vi "Calculate Ext Parameters.vi"(8 "error in":errorcluster, 11 "CRDS in":refnum<class "CRDS.lvclass">) -> (0 "error out":errorcluster, 2 "CRDS Data out":refnum<class "CRDS Data.lvclass">, 3 "CRDS out":refnum<class "CRDS.lvclass">)   [LabVIEW 2011, in "CRDS.lvclass"]
uses:
  CRDS.lvclass
  Data Class/Main Class/CRDS Data.lvclass
  Data Class/Cell Class/CRDS Cell Data.lvclass
  Cell Class/CRDS Cell.lvclass
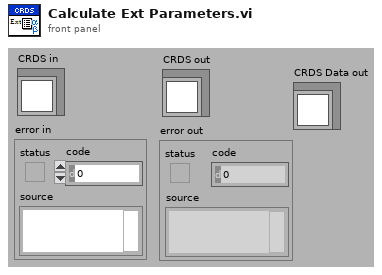
[diagram p1: front panel]
types:
  T1 = typedef "chDescr.ctl" = enum16{"Ref", "Dry", "60%", "90%"}
  T2 = typedef "las_lambda.ctl" = enum16{"Red", "Blue", "Green"}
  T3 = typedef "Get Tau Method.ctl" = enum8{"DFT-1", "DFT-5", "LRS"}
  T4 = cluster{"CalType":T3, "errorCalOn":bool, "lambda":sgl, "optTimeConst":sgl}
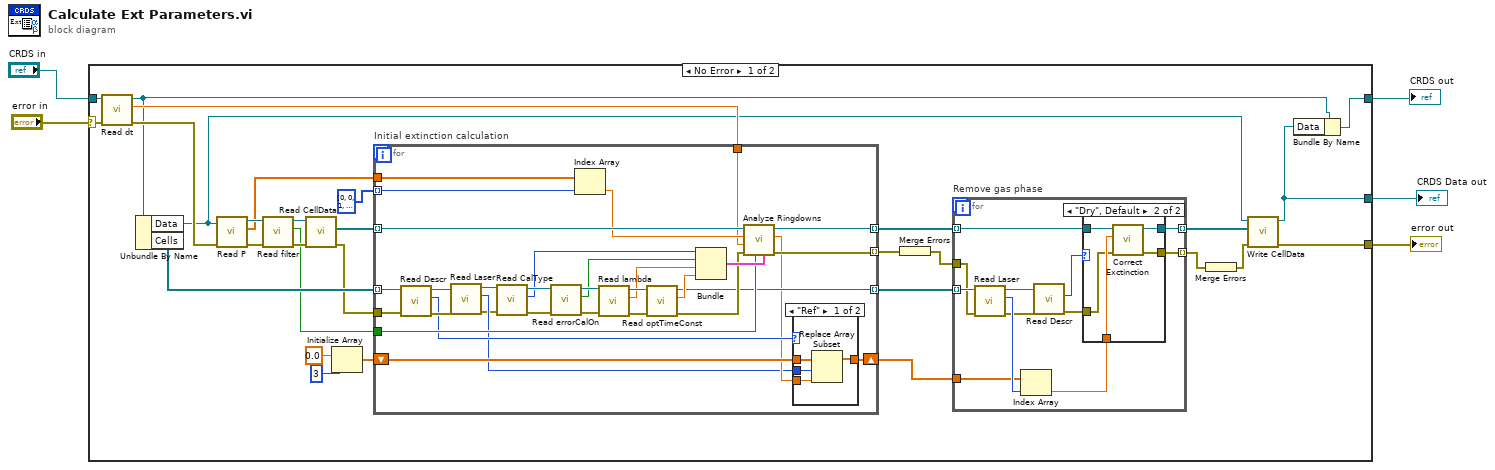
[diagram p0: block diagram]
diagram:
  n1 = case shown="No Error" "error in" {
    selector: "error in" -> [w23 w93]
    tunnel: [w10 w93] -> w4
    tunnel: [w8 w92] -> w2
    tunnel: "CRDS in" -> [w25 w92]
    tunnel: [w6 _] -> w1
    frame No Error {
      n2 = call "Read dt.vi"("error in (no error)"=w23, "CRDS in"=w25) -> ("error out"=w22:errorcluster, "dt"=w24:sgl, "CRDS out"=w9:refnum<class "CRDS.lvclass">)  [unwired: 7 in]
      n3 = Unbundle By Name(w9) -> ("Data"=w7:refnum<class "CRDS Data.lvclass">, "Cells"=w34:refnum<class "CRDS Cell.lvclass">[])
      n4 = call "Read P.vi"("error in (no error)"=w22, "CRDS Data in"=w7) -> ("error out"=w29:errorcluster, "P"=w26:sgl[], "CRDS Data out"=w28:refnum<class "CRDS Data.lvclass">)  [unwired: 7 in]
      n5 = call "Read filter.vi"("error in"=w29, "CRDS Data in"=w28) -> ("error out"=w31:errorcluster, "filter"=w30:bool, "CRDS Data out"=w32:refnum<class "CRDS Data.lvclass">)  [unwired: 7 in]
      n6 = call "Read CellData.vi"("error in"=w31, "CRDS Data in"=w32) -> ("error out"=w33:errorcluster, "CellData"=w35:refnum<class "CRDS Cell Data.lvclass">[])  [unwired: 7 in, 1 out]
      n7 = Initialize Array(sgl 0.0 ("element"), 3 ("dimension size")) -> (w15:sgl[])
      n8 = for "Initial extinction calculation" {
        tunnel: w35 -> [w86] mode=indexing
        tunnel: [w85] -> w20 mode=indexing
        tunnel: w34 -> [w65] mode=indexing
        tunnel: w33 -> [w64]
        tunnel: w30 -> [w73]
        tunnel: i32[] [0, 0, 1, 1, 1, 2, 2, 2] -> [w72] mode=indexing
        tunnel: w26 -> [w71]
        tunnel: w24 -> [w69]
        tunnel: [w67] -> w21 mode=indexing
        tunnel: [w66] -> w18 mode=indexing
        shift-right: [w59] -> w14
        shift-left: w15 -> [w61]
        n9 = call "Read Descr.vi"("error in (no error)"=w64, "CRDS Cell in"=w65) -> ("error out"=w62:errorcluster, "Descr"=w60:T1, "CRDS Cell out"=w63:refnum<class "CRDS Cell.lvclass">)  [unwired: 7 in]
        n10 = call "Read Laser.vi"("error in (no error)"=w62, "CRDS Cell in"=w63) -> ("error out"=w55:errorcluster, "Laser"=w57:T2, "CRDS Cell out"=w56:refnum<class "CRDS Cell.lvclass">)  [unwired: 7 in]
        n11 = call "Read CalType.vi"("error in (no error)"=w55, "CRDS Cell in"=w56) -> ("error out"=w84:errorcluster, "CalType"=w78:T3, "CRDS Cell out"=w83:refnum<class "CRDS Cell.lvclass">)  [unwired: 7 in]
        n12 = call "Read errorCalOn.vi"("error in (no error)"=w84, "CRDS Cell in"=w83) -> ("error out"=w82:errorcluster, "errorCalOn"=w77:bool, "CRDS Cell out"=w81:refnum<class "CRDS Cell.lvclass">)  [unwired: 7 in]
        n13 = Index Array(array=w71, index=w72) -> (element=w70:sgl)
        n14 = call "Read lambda.vi"("error in (no error)"=w82, "CRDS Cell in"=w81) -> ("error out"=w79:errorcluster, "lambda"=w76:sgl, "CRDS Cell out"=w80:refnum<class "CRDS Cell.lvclass">)  [unwired: 7 in]
        n15 = call "Read optTimeConst.vi"("error in (no error)"=w79, "CRDS Cell in"=w80) -> ("error out"=w68:errorcluster, "optTimeConst"=w75:sgl, "CRDS Cell out"=w66:refnum<class "CRDS Cell.lvclass">)  [unwired: 7 in]
        n16 = Bundle("CalType"=w78, "errorCalOn"=w77, "lambda"=w76, "optTimeConst"=w75) -> (w74:T4)  [unwired: 1 in]
        n17 = call "Analyze Ringdowns.vi"("CellData"=w74, "Filter?"=w73, "error in"=w68, "dt"=w69, "P"=w70, "CRDS Cell Data in"=w86) -> ("error out"=w67:errorcluster, "extCr"=w58:sgl, "CRDS Cell Data out"=w85:refnum<class "CRDS Cell Data.lvclass">)  [unwired: 3 in]
        n18 = case shown="\"Ref\"" w60 {
          tunnel: w61 -> [w90 w91]
          tunnel: [w87 w91] -> w59
          tunnel: w58 -> [w89 _]
          tunnel: w57 -> [w88 _]
          frame "Ref" {
            n19 = Replace Array Subset(array=w90, new element=w89, index=w88) -> (w87:sgl[])
          }
          frame "Dry", Default {
          }
        }
      }
      n20 = Merge Errors(w21) -> (w19:errorcluster)
      n21 = for "Remove gas phase" {
        tunnel: w20 -> [w44] mode=indexing
        tunnel: w19 -> [w40]
        tunnel: w18 -> [w47] mode=indexing
        tunnel: w14 -> [w42]
        tunnel: [w37] -> w12 mode=indexing
        tunnel: [w36] -> w13 mode=indexing
        n22 = call "Read Laser.vi"("error in (no error)"=w40, "CRDS Cell in"=w47) -> ("error out"=w39:errorcluster, "Laser"=w43:T2, "CRDS Cell out"=w46:refnum<class "CRDS Cell.lvclass">)  [unwired: 7 in]
        n23 = Index Array(array=w42, index=w43) -> (element=w41:sgl)
        n24 = call "Read Descr.vi"("error in (no error)"=w39, "CRDS Cell in"=w46) -> ("error out"=w38:errorcluster, "Descr"=w45:T1)  [unwired: 7 in, 1 out]
        n25 = case shown="\"Dry\", Default" w45 {
          tunnel: w44 -> [w49 w54]
          tunnel: w41 -> [_ w53]
          tunnel: w38 -> [w48 w52]
          tunnel: [w48 w51] -> w37
          tunnel: [w49 w50] -> w36
          frame "Ref" {
          }
          frame "Dry", Default {
            n26 = call "Correct Exctinction.vi"("error in"=w52, "refExt"=w53, "CRDS Cell Data in"=w54) -> ("error out"=w51:errorcluster, "CRDS Cell Data out"=w50:refnum<class "CRDS Cell Data.lvclass">)  [unwired: 7 in]
          }
        }
      }
      n27 = Merge Errors(w12) -> (w11:errorcluster)
      n28 = call "Write CellData.vi"("error in"=w11, "CellData"=w13, "CRDS Data in"=w7) -> ("error out"=w10:errorcluster, "CRDS Data out"=w6:refnum<class "CRDS Data.lvclass">)  [unwired: 7 in]
      n29 = Bundle By Name(cluster=w9, "Data"=w6) -> (w8:refnum<class "CRDS.lvclass">)
    }
    frame Error {
    }
  }
  "error out" <- w4
  "CRDS out" <- w2
  "CRDS Data out" <- w1
